vi "batch action return immediately.vi"() -> ()   [LabVIEW 2015]
uses:
  standard tasks/batch task/reporting type.ctl
  result/result.lvclass/result.ctl
  result/get data.vi
  result/get error.vi
  result/get data ID.vi
  result/get owning task.vi
  task/task.lvclass
  dispatcher/thread pool.lvclass
  standard reporters/event reporter/event reporter.lvclass
  result/result.lvclass
  standard tasks/batch task/batch task.lvclass
  standard action/wait action/wait action.lvclass
panel:
  out "x = y?":bool[](array[boolean])
  out "result names":string[](array[string])
  out "event times":u32[](array[numeric])
  out "iteration":i32
  out "errors":errorcluster[](array[cluster])
  out "data":variant[](array[variant])
  out "Time":u32
  out "error out":errorcluster
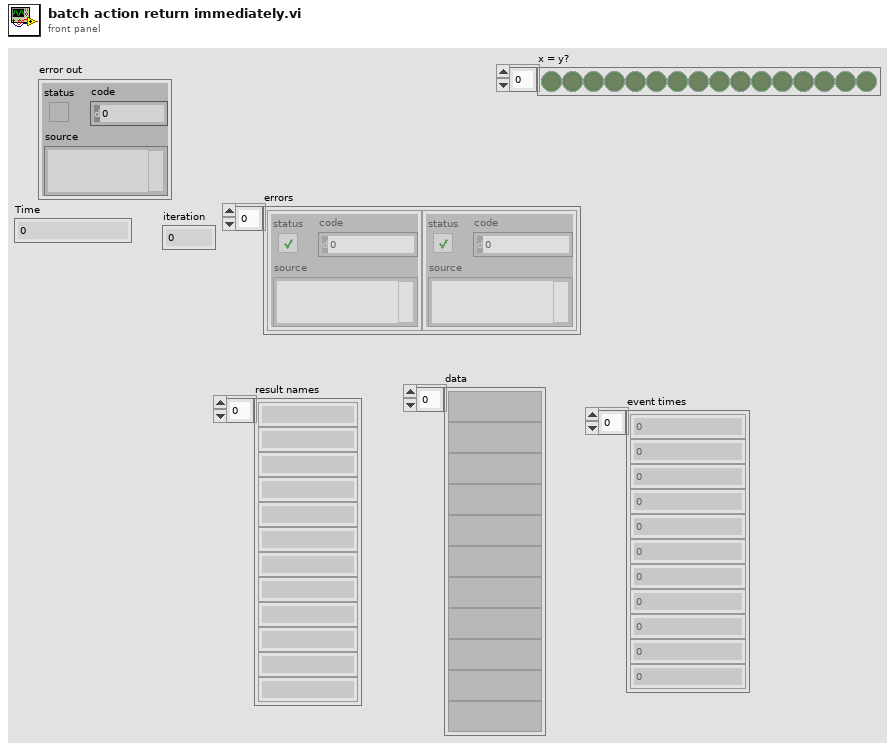
[diagram p1: front panel]
types:
  T1 = typedef "batch task.lvclass/reporting type.ctl" = enum16{"return immediately", "wait on all"}
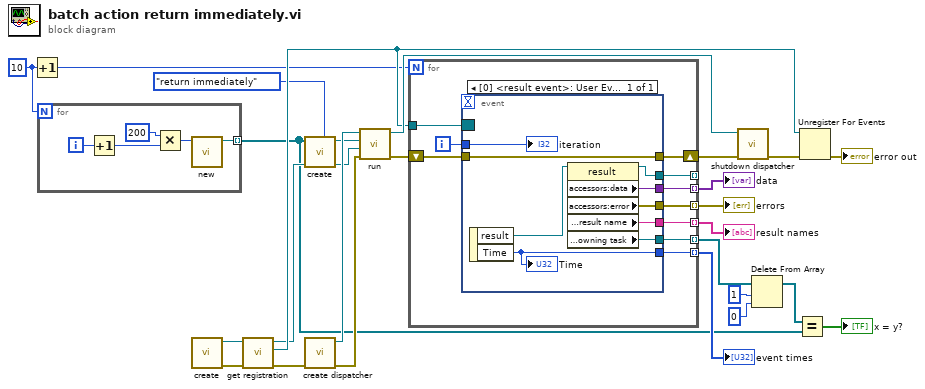
[diagram p0: block diagram]
diagram:
  w11 = 10 ("dimension size")
  n1 = Increment(x=w11) -> (x+1=w5:i32)
  n2 = for {
    N: w11 -> [_]
    tunnel: [w28] -> w7 mode=indexing
    i -> [w31]
    n3 = Increment(x=w31) -> (x+1=w30:i32)
    n4 = Multiply(x=200, y=w30) -> (x*y=w27:i32)
    n5 = call "new.vi"("timer"=w27) -> ("wait action out"=w28:refnum<class "wait action.lvclass">)  [unwired: 10 in]
  }
  n6 = call "create.vi"() -> ("error out"=w24:errorcluster, "event reporter out"=w25:refnum<class "event reporter.lvclass">)  [unwired: 10 in]
  n7 = call "get registration.vi"("error in"=w24, "event reporter in"=w25) -> ("error out"=w23:errorcluster, "result registration"=w16:refnum<event-registration>, "event reporter out"=w8:refnum<class "event reporter.lvclass">)  [unwired: 7 in]
  n8 = call "create.vi"("reporting type"=reporting_type."return immediately", "tasks"=w7) -> ("batch task out"=w17:refnum<class "batch task.lvclass">)  [unwired: 9 in]
  n9 = call "create dispatcher.vi"("error in"=w23) -> ("error out"=w9:errorcluster, "dispatcher"=w26:refnum<class "thread pool.lvclass">)  [unwired: 9 in]
  n10 = call "run.vi"("error in"=w9, "results reporter"=w8, "task"=w17, "thread pool in"=w26) -> ("error out"=w18:errorcluster, "thread pool out"=w22:refnum<class "thread pool.lvclass">)  [unwired: 6 in]
  n11 = for {
    N: w5 -> [_]
    tunnel: w16 -> [w41]
    shift-right: [w40] -> w19
    shift-left: w18 -> [w39]
    tunnel: [w38] -> w15 mode=indexing
    tunnel: [w37] -> w14 mode=indexing
    tunnel: [w36] -> _ mode=indexing
    tunnel: [w34] -> w13 mode=indexing
    tunnel: [w33] -> w10 mode=indexing
    tunnel: [w32] -> w3 mode=indexing
    i -> [w35]
    n12 = event shown="[0] <result event>: User Event" {
      selector: w41 -> [_]
      dyn-events: _ -> [_]
      timeout: _ -> [_]
      tunnel: [w50] -> w40
      tunnel: w39 -> [w50]
      tunnel: [w48] -> w38
      tunnel: [w47] -> w37
      tunnel: [w46] -> w36
      tunnel: w35 -> [w45]
      tunnel: [w44] -> w34
      tunnel: [w43] -> w33
      tunnel: [w42] -> w32
      event User Event {
        n13 = event-data() -> ("result"=w49:refnum<class "result.lvclass">, "Time"=w44:u32)  [unwired: 1 in]
        "Time" <- w44
        n14 = property class="result"(reference=w49) -> (reference out=w46:refnum<class "result.lvclass">, "accessors:data"=w48:variant, "accessors:error"=w47:errorcluster, "accessors:result name"=w43:string, "accessors:owning task"=w42:refnum<class "task.lvclass">)  [unwired: 1 in, 1 out]
        "iteration" <- w45
      }
    }
  }
  "data" <- w15
  "errors" <- w14
  "event times" <- w13
  "result names" <- w10
  n15 = call "shutdown dispatcher.vi"("error in"=w19, "thread pool"=w22) -> ("error out"=w21:errorcluster)  [unwired: 9 in]
  n16 = Delete From Array(array=w3, length=1, index=0) -> (array with subset deleted=w4:refnum<class "task.lvclass">[])  [unwired: 1 out]
  n17 = Equal?(x=w4, y=w7) -> (x = y?=→"x = y?":bool[])
  n18 = Unregister For Events(event registration refnum=w16, error in=w21) -> (error out=→"error out":errorcluster)
